vi "initializeArray.vi"(0 "Interior Points (1D)":cluster{"x":dbl, "y":dbl}[](array[cluster])) -> (1 "XMin":dbl, 2 "YMin":dbl, 4 "initialized array":dbl[][](array[numeric]))   [LabVIEW 2015]
panel:
  out "size(s)":i32[](array[numeric])
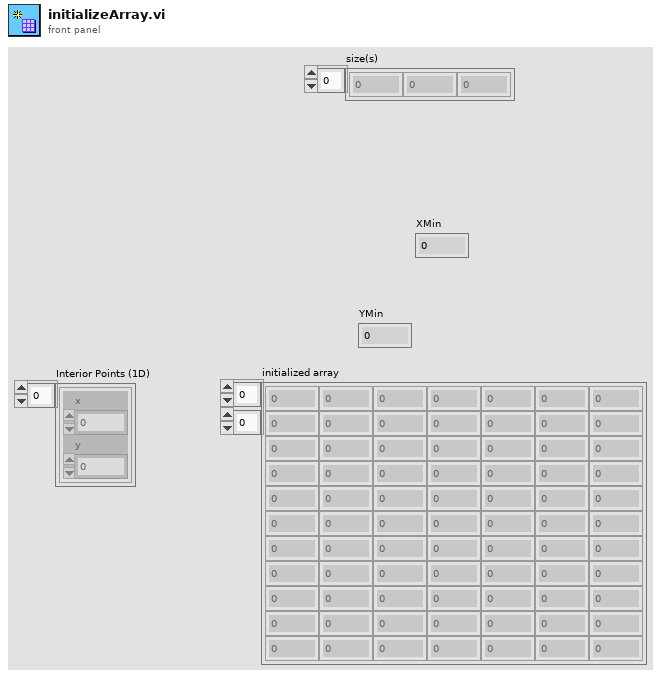
[diagram p1: front panel]
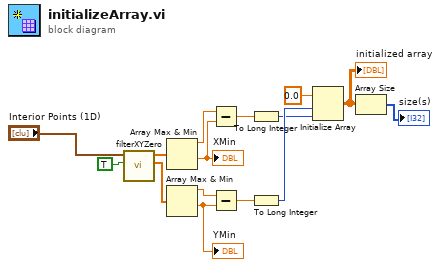
[diagram p0: block diagram]
diagram:
  n1 = call "filterXYZero.vi"("Filter Zero?"=TRUE, "Points"="Interior Points (1D)") -> ("Y"=w5:dbl[], "X"=w4:dbl[])  [unwired: 7 in, 1 out]
  n2 = Array Max & Min(array=w4) -> (max value=w13:dbl, min value=w8:dbl)  [unwired: 2 out]
  "XMin" <- w8
  n3 = Array Max & Min(array=w5) -> (max value=w14:dbl, min value=w7:dbl)  [unwired: 2 out]
  "YMin" <- w7
  n4 = Subtract(x=w13, y=w8) -> (x-y=w11:dbl)
  n5 = Subtract(x=w14, y=w7) -> (x-y=w12:dbl)
  n6 = To Long Integer(number=w11) -> (32bit integer=w9:i32)
  n7 = To Long Integer(number=w12) -> (32bit integer=w10:i32)
  n8 = Initialize Array(0.0 ("y"), w10, w9) -> (w2:dbl[][])
  "initialized array" <- w2
  n9 = Array Size(array=w2) -> (size(s)=→"size(s)":i32[])
